vi "Radau5_Initialization Check.vi"(11 "Simulation data":T1 {"Absolute tolerance" format="%.1e"; "Relative tolerance" format="%.1e"; "Output of T" format="%.1e"; "proposed step size" format="%.1e"; "min step size" format="%.1e"; "max step size" format="%.1e"; "final time" format="%.1e"; "step size" format="%.1e"; "initial time" format="%.1e"}) -> (3 "Simulation data out":T1 {"Absolute tolerance" format="%.1e"; "Relative tolerance" format="%.1e"; "Output of T" format="%.1e"; "proposed step size" format="%.1e"; "min step size" format="%.1e"; "max step size" format="%.1e"; "final time" format="%.1e"; "step size" format="%.1e"; "initial time" format="%.1e"})   [LabVIEW 2017, in "NI_DAE.lvlib"]
uses:
  <vilib>/gmath/NI_DAE.lvlib
  <vilib>/gmath/dae.llb/Radau5_Simulation Data.ctl
  <vilib>/gmath/dae.llb/Radau5_Diag Eval Stage.ctl
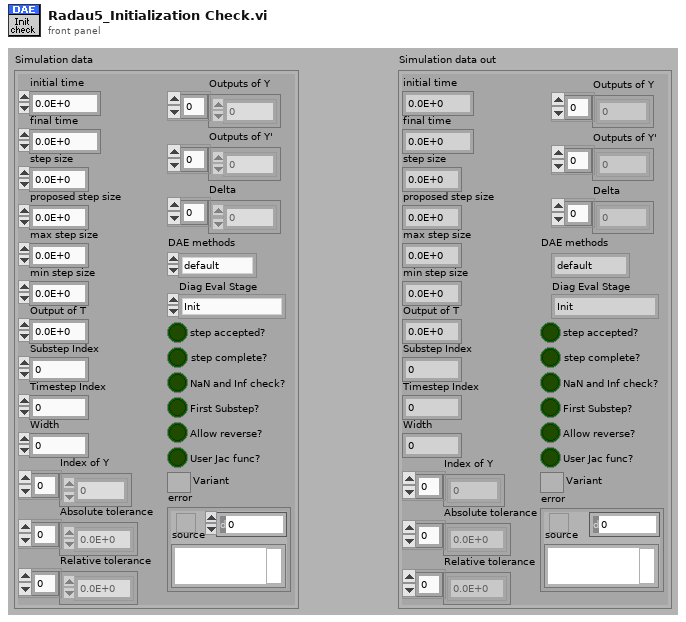
[diagram p1: front panel]
types:
  T1 = typedef "NI_DAE.lvlib/Radau5_Simulation Data.ctl" = cluster{"initial time":dbl, "final time":dbl, "step size":dbl, "proposed step size":dbl, "max step size":dbl, "min step size":dbl, "Output of T":dbl, "Substep Index":i32, "Timestep Index":i32, "Width":i32, "Absolute tolerance":dbl[], "Relative tolerance":dbl[], "Outputs of Y":dbl[], "Outputs of Y'":dbl[], "Delta":dbl[], "DAE methods":enum16{"default", "Radau IIA"}, "Diag Eval Stage":T2, "step accepted?":bool, "step complete?":bool, "NaN and Inf check?":bool, "First Substep?":bool, "Allow reverse?":bool, "error":errorcluster, "User Jac func?":bool, "Variant":variant, "Index of Y":i8[]}
  T2 = typedef "NI_DAE.lvlib/Radau5_Diag Eval Stage.ctl" = enum16{"Init", "Running", "Final", "End"}
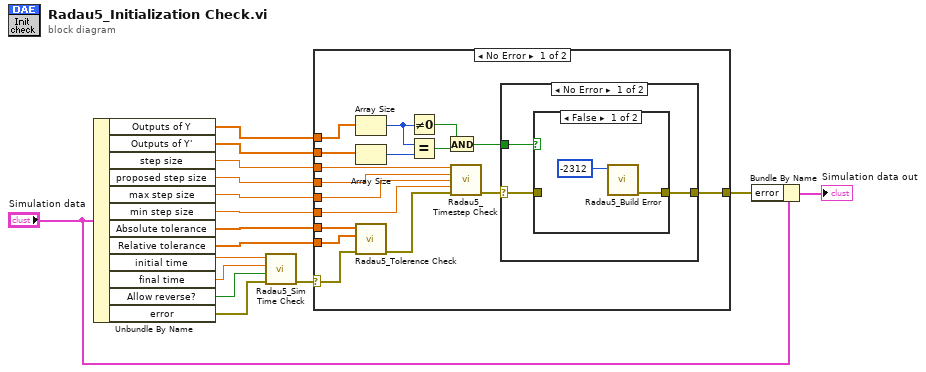
[diagram p0: block diagram]
diagram:
  n1 = Unbundle By Name("Simulation data") -> ("Outputs of Y"=w2:dbl[], "Outputs of Y'"=w1:dbl[], "step size"=w6:dbl, "proposed step size"=w7:dbl, "max step size"=w9:dbl, "min step size"=w8:dbl, "Absolute tolerance"=w5:dbl[], "Relative tolerance"=w4:dbl[], "initial time"=w13:dbl, "final time"=w14:dbl, "Allow reverse?"=w16:bool, "error"=w15:errorcluster)
  n2 = call <vilib>:"Radau5_Sim Time Check.vi"("error in (no error)"=w15, "Allow reverse?"=w16, "Final time"=w14, "Initial time"=w13) -> ("error out"=w12:errorcluster)  [unwired: 7 in]
  n3 = case shown="No Error" w12 {
    selector: w12 -> [w33 w41]
    tunnel: [w17 w41] -> w10
    tunnel: w9 -> [w27 _]
    tunnel: w8 -> [w26 _]
    tunnel: w7 -> [w28 _]
    tunnel: w6 -> [w29 _]
    tunnel: w5 -> [w32 _]
    tunnel: w4 -> [w31 _]
    tunnel: w2 -> [w25 _]
    tunnel: w1 -> [w24 _]
    frame No Error {
      n4 = Array Size(array=w25) -> (size(s)=w22:i32)
      n5 = Array Size(array=w24) -> (size(s)=w23:i32)
      n6 = call <vilib>:"Radau5_Tolerence Check.vi"("error in (no error)"=w33, "Absolute Tolerance"=w31, "Relative Tolerance"=w32) -> ("error out"=w30:errorcluster)  [unwired: 8 in]
      n7 = Not Equal To 0?(x=w22) -> (x != 0?=w21:bool)
      n8 = Equal?(x=w22, y=w23) -> (x = y?=w20:bool)
      n9 = And(x=w21, y=w20) -> (x .and. y?=w18:bool)
      n10 = call <vilib>:"Radau5_Timestep Check.vi"("time step"=w29, "Initial time step"=w28, "Max time step"=w27, "Min time step"=w26, "error in (no error)"=w30) -> ("error out"=w19:errorcluster)  [unwired: 10 in]
      n11 = case shown="No Error" w19 {
        selector: w19 -> [w35 w40]
        tunnel: w18 -> [w36 _]
        tunnel: [w34 w40] -> w17
        frame No Error {
          n12 = case shown="False" w36 {
            tunnel: w35 -> [_ w39]
            tunnel: [w37 w39] -> w34
            frame False {
              n13 = call <vilib>:"Radau5_Build Error.vi"("error code"=-2312 ("error.code")) -> ("error out"=w37:errorcluster)  [unwired: 10 in]
            }
            frame True {
            }
          }
        }
        frame Error {
        }
      }
    }
    frame Error {
    }
  }
  n14 = Bundle By Name(cluster="Simulation data", "error"=w10) -> (→"Simulation data out":T1)
